vi "Test_Create_Control.vi"   [LabVIEW 2025]
uses:
  8cebb4ce-4f0f-4319-9f7e-82e401bee674.vi
  0e244da9-745b-4f2d-a97c-0de3ccfbb071.vi
  57ba1f44-eecb-4af5-975d-0cda700306c1.vi
  Scripting Server.lvlib
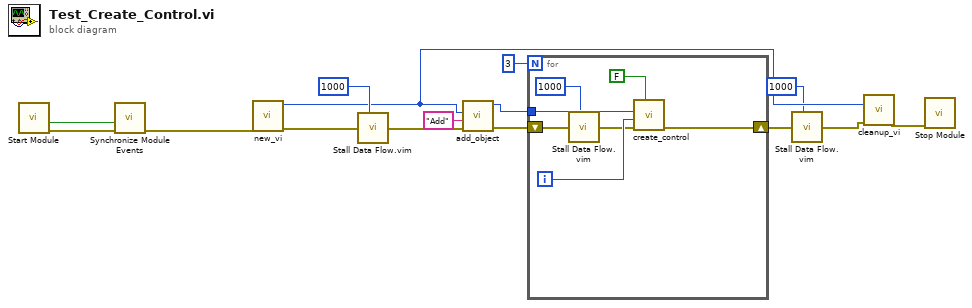
[diagram p0: block diagram]
diagram:
  n1 = call "Start Module.vi"() -> ("error out"=w14:errorcluster, "Wait for Event Sync?"=w15:bool)  [unwired: 7 in, 3 out]
  n2 = call "Synchronize Module Events.vi"("error in"=w14, "Wait for Event Sync?"=w15) -> ("error out"=w13:errorcluster)  [unwired: 9 in]
  n3 = call "new_vi.vi"("error in"=w13) -> ("error out"=w12:errorcluster, "vi_id"=w4:i32)  [unwired: 7 in, 2 out]
  n4 = call "Stall Data Flow.vim"("value in"=w12, "milliseconds to wait"=u32 1000) -> ("value out"=w11:errorcluster)  [unwired: 1 out]
  n5 = call "add_object.vi"("error in"=w11, "object_name"="Add", "vi_reference"=w4) -> ("error out"=w9:errorcluster, "object_id"=w8:i32)  [unwired: 5 in, 2 out]
  n6 = for {
    N: 3 -> [_]
    tunnel: w8 -> [w21]
    shift-right: [w17] -> w5
    shift-left: w9 -> [w22]
    i -> [w20]
    n7 = call "Stall Data Flow.vim"("value in"=w22, "milliseconds to wait"=u32 1000) -> ("value out"=w19:errorcluster)  [unwired: 1 out]
    n8 = call "create_control.vi"("constant"=FALSE, "error in"=w19, "terminal_index"=w20, "object_id"=w21) -> ("error out"=w17:errorcluster)  [unwired: 5 in, 2 out]
  }
  n9 = call "Stall Data Flow.vim"("value in"=w5, "milliseconds to wait"=u32 1000) -> ("value out"=w3:errorcluster)  [unwired: 1 out]
  n10 = call "cleanup_vi.vi"("error in"=w3, "vi_reference"=w4) -> ("error out"=w1:errorcluster)  [unwired: 7 in, 2 out]
  n11 = call "Stop Module.vi"("error in"=w1) -> ()  [unwired: 10 in, 1 out]
